vi "VALUE_EXCEEDED_CHECK.vi"(1 "Number of Channels":i32=5, 2 "Start Channel Index":i32, 3 "Max Value Array":dbl[](array[numeric]), 4 "Input Array":waveform(dbl)[](array[waveform])) -> (0 "Array":bool[](array[boolean]))   [LabVIEW 2013]
doc: "Checks if any values in an incoming array of waveforms exceed a corresponding maximum value."
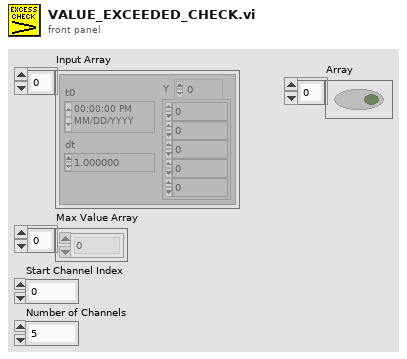
[diagram p1: front panel]
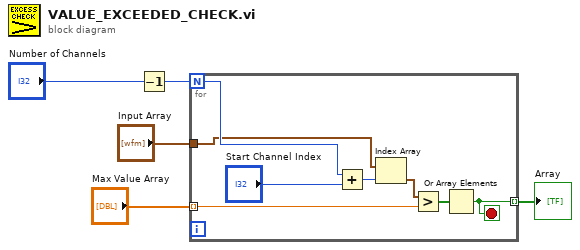
[diagram p0: block diagram]
diagram:
  n1 = Decrement(x="Number of Channels") -> (x-1=w1:i32)
  n2 = for {
    N: w1 -> [w11]
    tunnel: [w12] -> w3 mode=indexing
    tunnel: "Max Value Array" -> [w10] mode=indexing
    tunnel: "Input Array" -> [w9]
    stop <- w12 stop-if-true
    n3 = Add(x=w11, y="Start Channel Index") -> (x+y=w6:i32)
    n4 = Index Array(array=w9, index=w6) -> (element=w8:waveform(dbl))
    n5 = Greater?(x=w8, y=w10) -> (0:w13:bool[])
    n6 = Or Array Elements(Boolean array=w13) -> (logical OR=w12:bool)
  }
  "Array" <- w3
